vi "Bert_or_Ernie.vi"() -> ()   [LabVIEW 2015]
panel:
  in  "On Comp?":bool
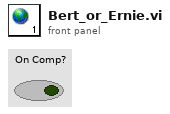
[diagram p1: front panel]
diagram:
